vi "Set Current.vi"(8 "error in (no error)":errorcluster, 10 "Setpoint In":dbl, 11 "Reload-pro in":refnum<class "Reload-pro.lvclass">) -> (0 "error out":errorcluster, 2 "Setpoint Out":dbl, 3 "Reload-pro out":refnum<class "Reload-pro.lvclass">)   [LabVIEW 2013, in "Reload-pro.lvclass"]
uses:
  Reload-pro.lvclass
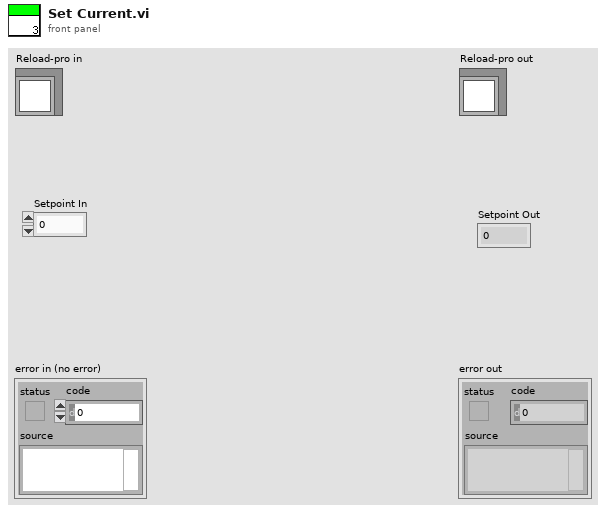
[diagram p1: front panel]
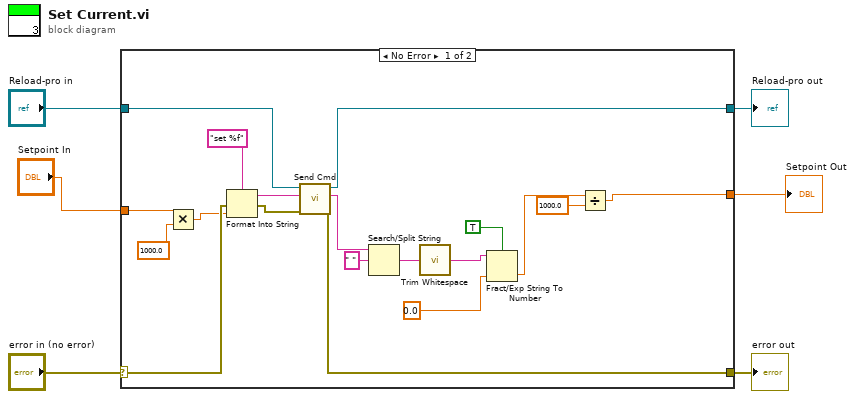
[diagram p0: block diagram]
diagram:
  n1 = case shown="No Error" "error in (no error)" {
    selector: "error in (no error)" -> [w16 w27]
    tunnel: [w21 w27] -> w5
    tunnel: [w19 w26] -> w3
    tunnel: "Reload-pro in" -> [w20 w26]
    tunnel: [w10 _] -> w2
    tunnel: "Setpoint In" -> [w9 _]
    frame No Error {
      n2 = Multiply(x=w9, y=1000.0) -> (x*y=w8:dbl)
      n3 = Format Into String(format string="set %f", error in=w16, w8) -> (resulting string=w18:string, error out=w15:errorcluster)  [unwired: 1 in]
      n4 = call-dynamic "Send Cmd.vi"("error in (no error)"=w15, "Command"=w18, "Reload-pro in"=w20) -> ("error out"=w21:errorcluster, "Response"=w25:string, "Reload-pro out"=w19:refnum<class "Reload-pro.lvclass">)  [unwired: 6 in]
      n5 = Search/Split String(string=w25, search string/char (-)=" ") -> (match + rest of string=w23:string)  [unwired: 1 in, 2 out]
      n6 = call <vilib>:"Trim Whitespace.vi"("string"=w23) -> ("trimmed string"=w14:string)  [unwired: 1 in]
      n7 = Fract/Exp String To Number(use system decimal point (T)=TRUE, string=w14, default (0 dbl)=0.0) -> (number=w12:dbl)  [unwired: 1 in, 1 out]
      n8 = Divide(x=w12, y=1000.0) -> (x/y=w10:dbl)
    }
    frame Error {
    }
  }
  "error out" <- w5
  "Reload-pro out" <- w3
  "Setpoint Out" <- w2
